vi "HORNDOWN.vi"() -> ()   [LabVIEW 2017]
panel:
  out "mm":u8
  out "N":u8
  out "mm pre":dbl
  out "inch pre":dbl
  out "inch":dbl
  out "mm":dbl
  # "ACTUATOR SETUP :  HORN DOWN"
  # "Actual distance"
  # "Actual force"
  # "Absolute distance"
  # "PrePartContact"
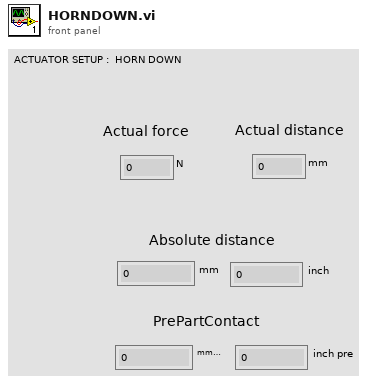
[diagram p1: front panel]
types:
  T1 = enum16{"big-endian, network order", "native, host order", "little-endian"}
  T2 = enum16{"Standard", "Buffered", "CRLF", "Immediate"}
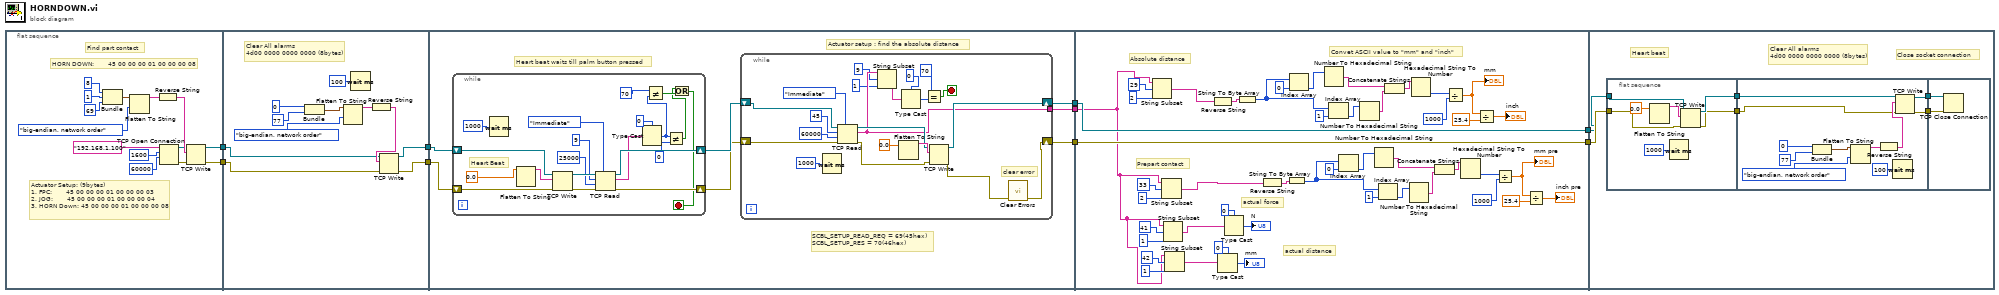
[diagram p0: block diagram]
diagram:
  n1 = flat-sequence {
    tunnel: [w16] -> w4
    tunnel: [w15] -> w2
    tunnel: w4 -> [w27]
    tunnel: [w25] -> w3
    tunnel: w2 -> [w26]
    tunnel: [w24] -> w1
    tunnel: w3 -> [w41]
    tunnel: w1 -> [w40]
    tunnel: [w39] -> w9
    tunnel: [w38] -> w8
    tunnel: [w35] -> w7
    tunnel: w9 -> [w114]
    tunnel: w8 -> [w115]
    tunnel: w7 -> [w89]
    tunnel: [w115] -> w6
    tunnel: [w114] -> w5
    tunnel: w6 -> [w135]
    tunnel: w5 -> [w134]
    frame #0 {
      # "Actuator Setup: (9bytes)\n1. FPC:       45 00 00 00 01 00 00 00 03\n2. JOG:       45 00 00 00 01 00 00 00 04\n3. HORN Down: 45 00 00 00 01 00 00 00 08"
      # "Find part contact"
      # "HORN DOWN:       45 00 00 00 01 00 00 00 08"
      n2 = Bundle(i8 8, 1, 69) -> (w12:cluster{i8, i32, i32})  [unwired: 1 in]
      n3 = Flatten To String(anything=w12, byte order (0:big-endian, network order)=T1."big-endian, network order") -> (data string=w23:string)  [unwired: 2 in, 2 out]
      n4 = Reverse String(1:w23) -> (0:w22:string)
      n5 = TCP Open Connection(address="192.168.1.100", remote port or service name=u16 1600, timeout ms (60000)=60000) -> (connection ID=w21:refnum<k5>, error out=w20:errorcluster)  [unwired: 2 in]
      n6 = TCP Write(connection ID=w21, data in=w22, error in (no error)=w20) -> (connection ID out=w16:refnum<k5>, error out=w15:errorcluster)  [unwired: 1 in, 1 out]
    }
    frame #1 {
      # "Clear All alarms\n4d00 0000 0000 0000 (8bytes)"
      n7 = Bundle(0, 77) -> (w34:cluster{i32, i32})  [unwired: 1 in]
      n8 = Flatten To String(anything=w34, byte order (0:big-endian, network order)=T1."big-endian, network order") -> (data string=w33:string)  [unwired: 2 in, 2 out]
      n9 = Wait (ms)(milliseconds to wait=u32 100) -> ()  [unwired: 1 out]
      n10 = Reverse String(1:w33) -> (0:w29:string)
      n11 = TCP Write(connection ID=w27, data in=w29, error in (no error)=w26) -> (connection ID out=w25:refnum<k5>, error out=w24:errorcluster)  [unwired: 1 in, 1 out]
    }
    frame #2 {
      # "SCBL_SETUP_READ_REQ = 69(45hex)\nSCBL_SETUP_RES = 70(46hex)"
      # "Actuator setup : find the absolute distance"
      # "Heart beat waits till palm button pressed"
      n12 = while {
        shift-right: [w59] -> w37
        shift-left: w41 -> [w61]
        shift-right: [w58] -> w36
        shift-left: w40 -> [w60]
        stop <- w46 stop-if-true
        # "Heart Beat"
        n13 = Wait (ms)(milliseconds to wait=u32 1000) -> ()  [unwired: 1 out]
        n14 = Flatten To String(anything=0.0) -> (data string=w56:string)  [unwired: 3 in, 2 out]
        n15 = TCP Write(connection ID=w61, data in=w56, error in (no error)=w60) -> (connection ID out=w55:refnum<k5>, error out=w54:errorcluster)  [unwired: 1 in, 1 out]
        n16 = TCP Read(connection ID=w55, bytes to read=9, error in (no error)=w54, 7:T2."Immediate" ("mode (standard)"), 9:25000 ("timeout ms (25000)")) -> (connection ID out=w59:refnum<k5>, data out=w49:string, error out=w58:errorcluster)
        n17 = Type Cast(type=u8 0, x=w49) -> (*(type *) &x=w42:u8)
        n18 = Not Equal?(x=u8 70, y=w42) -> (x != y?=w45:bool)
        n19 = Not Equal?(x=w42, y=u8 0) -> (x != y?=w44:bool)
        n20 = Or(x=w44, y=w45) -> (x .or. y?=w46:bool)
      }
      n21 = while {
        tunnel: [w68] -> w35
        shift-right: [w70] -> w39
        shift-left: w37 -> [w82]
        shift-right: [w69] -> w38
        shift-left: w36 -> [w81]
        stop <- w76 stop-if-true
        # "clear error"
        n22 = Wait (ms)(milliseconds to wait=u32 1000) -> ()  [unwired: 1 out]
        n23 = TCP Read(connection ID=w82, bytes to read=45, error in (no error)=w81, 7:T2."Immediate" ("mode (standard)"), 9:60000 ("timeout ms (25000)")) -> (connection ID out=w73:refnum<k5>, data out=w68:string, error out=w72:errorcluster)
        n24 = String Subset(string=w68, offset (0)=9, length (rest)=1 ("length (rest)")) -> (substring=w63:string)
        n25 = Flatten To String(anything=0.0) -> (data string=w74:string)  [unwired: 3 in, 2 out]
        n26 = Type Cast(type=u8 0, x=w63) -> (*(type *) &x=w65:u8)
        n27 = Equal?(x=u8 70, y=w65) -> (x = y?=w76:bool)
        n28 = TCP Write(connection ID=w73, data in=w74, error in (no error)=w72) -> (connection ID out=w70:refnum<k5>, error out=w71:errorcluster)  [unwired: 1 in, 1 out]
        n29 = call <vilib>:"Clear Errors.vi"("error in (no error)"=w71) -> ("error out"=w69:errorcluster)  [unwired: 5 in, 1 out]
      }
    }
    frame #3 {
      # "actual distance"
      # "actual force"
      # "Convet ASCII value to \"mm\" and \"inch\""
      # "Prepart contact"
      # "Absolute distance"
      n30 = String Subset(string=w89, offset (0)=29, length (rest)=2 ("length (rest)")) -> (substring=w127:string)
      n31 = String Subset(string=w89, offset (0)=33, length (rest)=2 ("length (rest)")) -> (substring=w94:string)
      n32 = String Subset(string=w89, offset (0)=41, length (rest)=1 ("length (rest)")) -> (substring=w88:string)
      n33 = String Subset(string=w89, offset (0)=42, length (rest)=1 ("length (rest)")) -> (substring=w83:string)
      n34 = Reverse String(1:w127) -> (0:w126:string)
      n35 = Type Cast(type=u8 0, x=w83) -> (*(type *) &x=→"mm":u8)
      n36 = Type Cast(type=u8 0, x=w88) -> (*(type *) &x=→"N":u8)
      n37 = String To Byte Array(string=w126) -> (unsigned byte array=w121:u8[])
      n38 = Reverse String(1:w94) -> (0:w95:string)
      n39 = String To Byte Array(string=w95) -> (unsigned byte array=w100:u8[])
      n40 = Index Array(array=w121, index=0) -> (element=w124:u8)
      n41 = Number To Hexadecimal String(2:w124) -> (0:w119:string)  [unwired: 1 in]
      n42 = Index Array(array=w121, index=1) -> (element=w123:u8)
      n43 = Index Array(array=w100, index=0) -> (element=w97:u8)
      n44 = Number To Hexadecimal String(2:w123) -> (0:w120:string)  [unwired: 1 in]
      n45 = Number To Hexadecimal String(2:w97) -> (0:w102:string)  [unwired: 1 in]
      n46 = Index Array(array=w100, index=1) -> (element=w98:u8)
      n47 = Concatenate Strings(w119, w120) -> (w118:string)
      n48 = Number To Hexadecimal String(2:w98) -> (0:w101:string)  [unwired: 1 in]
      n49 = Hexadecimal String To Number(string=w118) -> (number=w117:u32)  [unwired: 2 in, 1 out]
      n50 = Concatenate Strings(w102, w101) -> (w103:string)
      n51 = Divide(x=w117, y=1000) -> (x/y=w113:dbl)
      "mm" <- w113
      n52 = Hexadecimal String To Number(string=w103) -> (number=w104:u32)  [unwired: 2 in, 1 out]
      n53 = Divide(x=w113, y=25.4) -> (x/y=→"inch":dbl)
      n54 = Divide(x=w104, y=1000) -> (x/y=w106:dbl)
      "mm pre" <- w106
      n55 = Divide(x=w106, y=25.4) -> (x/y=→"inch pre":dbl)
    }
    frame #4 {
      # "Clear All alarms\n4d00 0000 0000 0000 (8bytes)"
      # "Close socket connection"
      # "Heart beat"
      n56 = flat-sequence {
        tunnel: w135 -> [w137]
        tunnel: w134 -> [w139]
        tunnel: [w138] -> w133
        tunnel: [w136] -> w131
        tunnel: w133 -> [w147]
        tunnel: [w145] -> w132
        tunnel: w131 -> [w146]
        tunnel: [w144] -> w130
        tunnel: w132 -> [w155]
        tunnel: w130 -> [w154]
        frame #0 {
          n57 = Flatten To String(anything=0.0) -> (data string=w140:string)  [unwired: 3 in, 2 out]
          n58 = Wait (ms)(milliseconds to wait=u32 1000) -> ()  [unwired: 1 out]
          n59 = TCP Write(connection ID=w139, data in=w140, error in (no error)=w137) -> (connection ID out=w138:refnum<k5>, error out=w136:errorcluster)  [unwired: 1 in, 1 out]
        }
        frame #1 {
          n60 = Bundle(0, 77) -> (w153:cluster{i32, i32})  [unwired: 1 in]
          n61 = Flatten To String(anything=w153, byte order (0:big-endian, network order)=T1."big-endian, network order") -> (data string=w152:string)  [unwired: 2 in, 2 out]
          n62 = Reverse String(1:w152) -> (0:w148:string)
          n63 = Wait (ms)(milliseconds to wait=u32 100) -> ()  [unwired: 1 out]
          n64 = TCP Write(connection ID=w147, data in=w148, error in (no error)=w146) -> (connection ID out=w145:refnum<k5>, error out=w144:errorcluster)  [unwired: 1 in, 1 out]
        }
        frame #2 {
          n65 = TCP Close Connection(connection ID=w155, error in (no error)=w154) -> ()  [unwired: 1 in, 2 out]
        }
      }
    }
  }
